vi "Switch_heater.vi"(2 "Boolesch":bool=TRUE, 3 "PSU Setup":T1={"Max Sweep(4.2K)"=0.003516666666666667, "Max Sweep(2.2K)"=0.003516666666666667, "Switch htr dly"=60.0, "O/P contactor?"=FALSE, "Max Field(4.2K)"=0.211, "Max Field(2.2K)"=0.211, "Description\n"="", "Settings.vi"=path "", "Max lead res"=0.5, "IO Info"={"Address"={"Com Port"=1, "ISOBUS Address"=1, "GPIB Address"=24, "Communication"=enum."ISOBUS"}, "Version"=enum."IPS"}, "Adjust shims"=FALSE} {"Max lead res" format="%.2f"; "Max Field(2.2K)" format="%.2f"; "Max Field(4.2K)" format="%.2f"; "Switch htr dly" format="%.2f"; "Max Sweep(2.2K)" format="%.2f"; "Max Sweep(4.2K)" format="%.2f"}) -> ()   [LabVIEW 2016]
uses:
  Oxford Software/Oxsoft/PSAPPS.LLB/PSSetup.ctl
  Oxford Software/Oxsoft/PSSUBS.LLB/PSIO.ctl
  Oxford Software/Oxsoft/BUSGEN.LLB/OxfordAddress.ctl
  Global/Global Variables/Data_Display_global.vi
panel:
  out "Select 2":bool
  # "Press Shift F1 to edit this field"
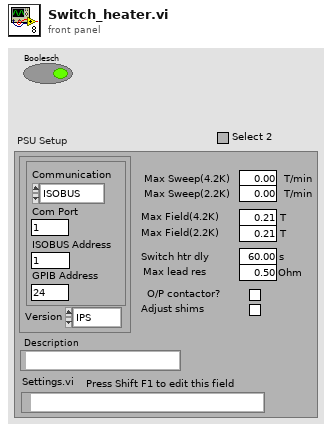
[diagram p1: front panel]
types:
  T1 = typedef "PSSetup.ctl" = cluster{"Max Sweep(4.2K)":dbl[unit], "Max Sweep(2.2K)":dbl[unit], "Switch htr dly":dbl[unit], "O/P contactor?":bool, "Max Field(4.2K)":dbl[unit], "Max Field(2.2K)":dbl[unit], "Description\n":string, "Settings.vi":path, "Max lead res":dbl[unit], "IO Info":T2, "Adjust shims":bool}
  T2 = typedef "PSIO.ctl" = cluster{"Address":T3, "Version":enum16{"PS", "IPS"}}
  T3 = typedef "OxfordAddress.ctl" = cluster{"Com Port":i32, "ISOBUS Address":i32, "GPIB Address":i16, "Communication":enum16{"RS232", "ISOBUS", "GPIB", "Gateway"}}
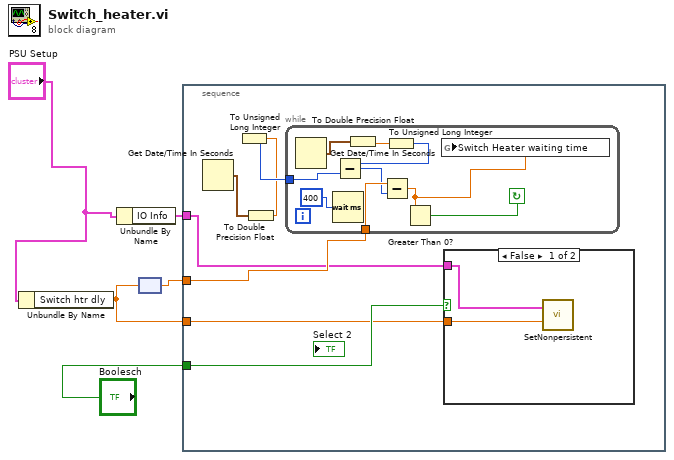
[diagram p0: block diagram]
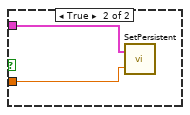
[diagram p2: hidden frame]
diagram:
  n1 = Unbundle By Name("PSU Setup") -> ("Switch htr dly"=w1:dbl[unit])
  n2 = Unbundle By Name("PSU Setup") -> ("IO Info"=w2:T2)
  n3 = node(w1) -> (w4:dbl)
  n4 = stacked-sequence {
    tunnel: w4 -> [w8]
    tunnel: "Boolesch" -> [w9]
    tunnel: w2 -> [w7]
    tunnel: w1 -> [w6]
    frame #0 {
      n5 = Get Date/Time In Seconds() -> (seconds since 1Jan1904=w10:timestamp)
      n6 = To Double Precision Float(number=w10) -> (double precision float=w11:dbl)
      n7 = To Unsigned Long Integer(number=w11) -> (unsigned 32bit integer=w12:u32)
      n8 = while {
        tunnel: w8 -> [w19]
        tunnel: w12 -> [w20]
        stop <- w14 continue-if-true
        n9 = Get Date/Time In Seconds() -> (seconds since 1Jan1904=w16:timestamp)
        n10 = Wait (ms)(milliseconds to wait=u32 400) -> ()  [unwired: 1 out]
        n11 = To Double Precision Float(number=w16) -> (double precision float=w17:dbl)
        n12 = To Unsigned Long Integer(number=w17) -> (unsigned 32bit integer=w21:u32)
        n13 = Subtract(x=w21, y=w20) -> (x-y=w15:u32)
        n14 = Subtract(x=w19, y=w15) -> (x-y=w13:dbl)
        n15 = Greater Than 0?(x=w13) -> (x > 0?=w14:bool)
        n16 = global write "Data_Display_global.vi" "Switch Heater waiting time"(w13) -> ()
      }
      n17 = case shown="False" w9 {
        tunnel: w7 -> [w23 w25]
        tunnel: w6 -> [w22 w24]
        frame False {
          n18 = call "SetNonpersistent.vi"("Switch Heater Dwell Time"=w22, "IO Info"=w23) -> ()  [unwired: 2 out]
        }
        frame True {
          n19 = call "SetPersistent.vi"("Switch Heater Dwell Time"=w24, "IO Info"=w25) -> ()  [unwired: 1 in, 1 out]
        }
      }
    }
  }
